vi "SetVoltage_MultiVoltageSource.vi"(8 "error in (no error)":errorcluster, 9 "Channel Value":dbl=0.2, 10 "Channel":i32=1, 11 "VISA Refnum in":refnum<visa-resource-name>) -> (0 "error out":errorcluster, 3 "VISA Refnum out":refnum<visa-resource-name>)   [LabVIEW 2020]
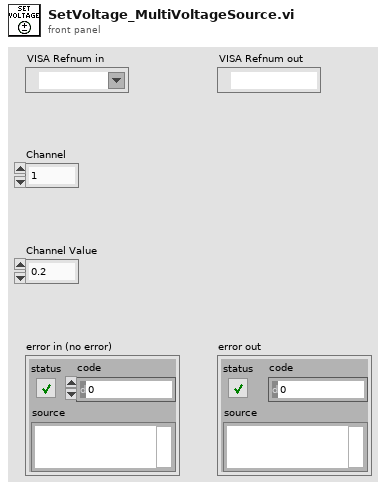
[diagram p1: front panel]
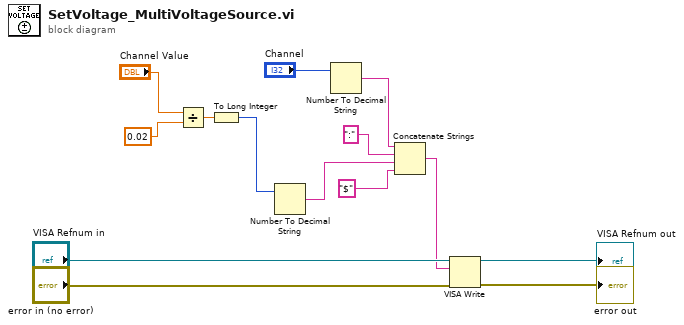
[diagram p0: block diagram]
diagram:
  n1 = Divide(x="Channel Value", y=0.02) -> (x/y=w2:dbl)
  n2 = To Long Integer(number=w2) -> (32bit integer=w4:i32)
  n3 = Number To Decimal String(number=w4) -> (decimal integer string=w1:string)  [unwired: 1 in]
  n4 = Number To Decimal String(number="Channel") -> (decimal integer string=w9:string)  [unwired: 1 in]
  n5 = Concatenate Strings(w9, ":" ("string"), w1, "$" ("string")) -> (w5:string)
  n6 = VISA Write(VISA resource name="VISA Refnum in", write buffer=w5, error in (no error)="error in (no error)") -> (VISA resource name out=→"VISA Refnum out":refnum<visa-resource-name>, error out=→"error out":errorcluster)  [unwired: 1 out]
